vi "Fire User Event.vi"(8 "error in (no error)":errorcluster, 11 "User Event":refnum<user-event>) -> (0 "error out":errorcluster)   [LabVIEW 2015, in "User Events.lvlib"]
uses:
  User Events.lvlib
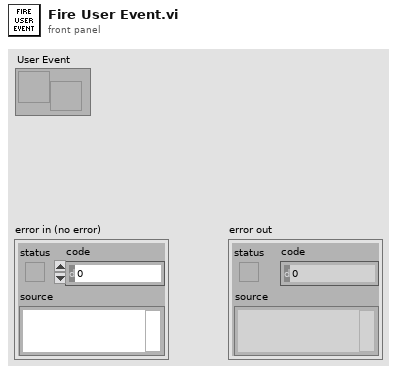
[diagram p1: front panel]
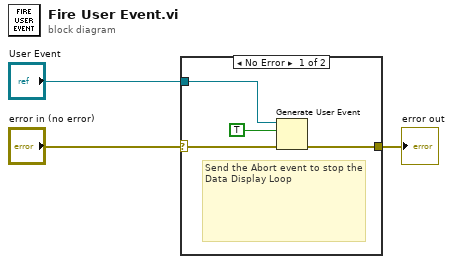
[diagram p0: block diagram]
diagram:
  n1 = case shown="No Error" "error in (no error)" {
    selector: "error in (no error)" -> [w4 w8]
    tunnel: [w6 w8] -> w3
    tunnel: "User Event" -> [w5 _]
    frame No Error {
      # "Send the Abort event to stop the Data Display Loop"
      n2 = Generate User Event(user event=w5, event data cluster=TRUE ("event data"), error in=w4) -> (error out=w6:errorcluster)  [unwired: 1 in, 1 out]
    }
    frame Error {
    }
  }
  "error out" <- w3
